vi "Initialize Buffer IDs.vi"(8 "error in":errorcluster, 10 "shared resources":refnum<class "Shared Resources.lvclass">, 11 "rx execution unit":refnum<class "Rx Execution Unit.lvclass">) -> (0 "error out":errorcluster, 3 "rx execution unit out":refnum<class "Rx Execution Unit.lvclass">)   [LabVIEW 2020, in "AIM MIL-STD-1553 Engine.lvlib" / "Implementation.lvlib" / "Rx Execution Unit.lvclass"]
uses:
  Rx Execution Unit.lvclass
  Interfaces/Shared Resources/Shared Resources.lvclass
  Shared Resources/Shared Resources.lvclass
  Shared Resources/Shared Resources.lvclass/Shared Resources.ctl
  Rx Execution Unit.lvclass/Rx Execution Unit.ctl
  Shared/Direction.ctl
  Shared Resources/Read BC Subaddress to Buffer ID Map.vi
  Shared Resources/Read RT Subaddress to Buffer ID Map.vi
  <vilib>/NI VeriStand/Custom Device Tools/Custom Device Utility Library/Custom Device Utility Library.lvlib
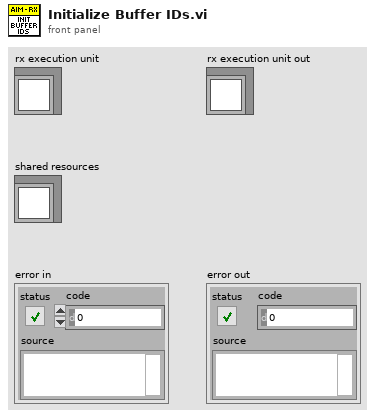
[diagram p1: front panel]
types:
  T1 = enum16{"unknown", "BC Message Buffer", "RT Message Buffer"}
  T2 = typedef "Direction.ctl" = enum16{"Rx", "Tx"}
  T3 = typedef "AIM MIL-STD-1553 Engine.lvlib/Implementation.lvlib/Shared Resources.lvclass/BC Subaddress to Buffer ID Map.ctl" = map{cluster{"TX Address":u8, "TX Subaddress":u8, "RX Address":u8, "RX Subaddress":u8}, cluster{"Buffer ID":u16}}
  T4 = typedef "AIM MIL-STD-1553 Engine.lvlib/Implementation.lvlib/Shared Resources.lvclass/RT Subaddress to Buffer ID Map.ctl" = map{cluster{"RT Address":u8, "Subaddress":u8, "Direction":T2}, cluster{"Buffer ID":u16}}
  T5 = typedef "AIM MIL-STD-1553 Engine.lvlib/Custom Device.lvlib/Compiled Message.ctl" = cluster{"Message Section Handle":T6, "First Parameter Index":i32, "Parameter Channel Handles":T6[], "Direction":T2, "Parameters":T7[], "Receiving RT Address":u8, "Receiving RT Sub-address":u8, "Transmitting RT Address":u8, "Transmitting RT Sub-address":u8, "Word Count":u8, "Buffer Type":enum16{"unknown", "BC Message Buffer", "RT Message Buffer"}, "Buffer ID":u16, "Terminal Type":enum16{"Bus Controller", "Remote Terminal"}, "Timestamp Enabled":bool, "Timestamp Channel Handle":T6}
  T6 = typedef "Custom Device API.lvlib/Custom Device Item Ref.ctl" = u64
  T7 = typedef "Parameter Definition.ctl" = cluster{"start index":i32, "size (bits)":i32, "encoding":enum16{"BNR", "BCD", "Discrete"}, "signed":bool, "multiplier":dbl, "offset":dbl}
  T8 = cluster{"Receiving RT Address":u8, "Receiving RT Sub-address":u8, "Direction":T2}
  T9 = cluster{"Transmitting RT Address":u8, "Transmitting RT Sub-address":u8, "Receiving RT Address":u8, "Receiving RT Sub-address":u8}
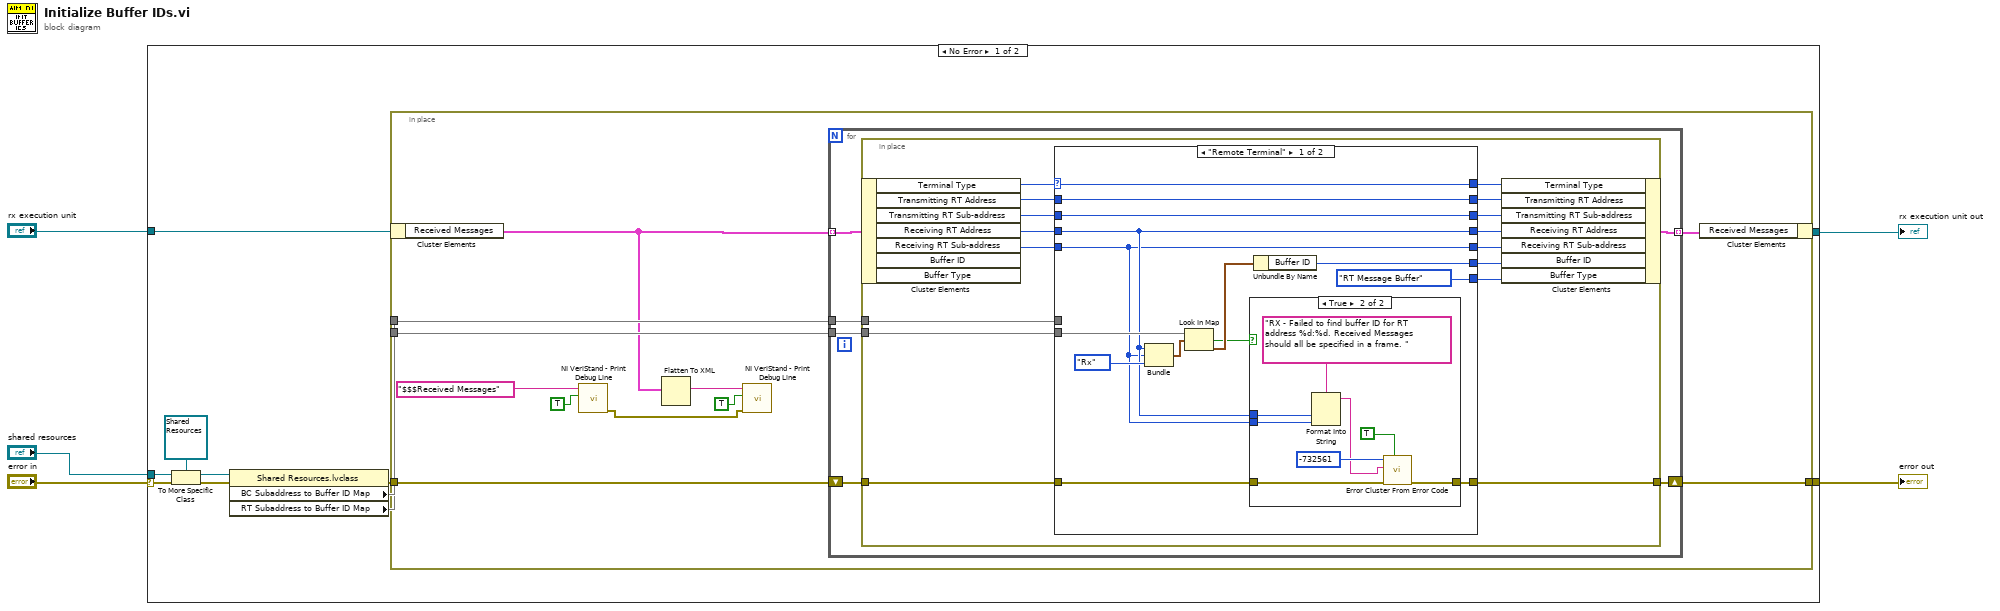
[diagram p0: block diagram]
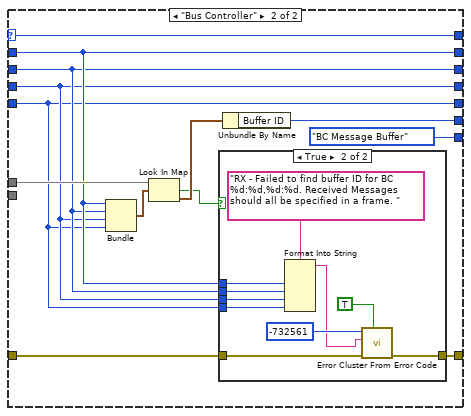
[diagram p3: hidden frame]
diagram:
  n1 = case shown="No Error" "error in" {
    selector: "error in" -> [w16 w98]
    tunnel: "shared resources" -> [w15 _]
    tunnel: [w11 w98] -> w4
    tunnel: "rx execution unit" -> [w10 w97]
    tunnel: [w9 w97] -> w2
    frame No Error {
      n2 = To More Specific Class(target class=refnum<class "Shared Resources.lvclass"> refnum ("specific class reference"), reference=w15, error in=w16) -> (specific class reference=w12:refnum<class "Shared Resources.lvclass">, error out=w6:errorcluster)
      n3 = property class="Shared Resources.lvclass"(reference=w12, error in=w6) -> (error out=w13:errorcluster, "BC Subaddress to Buffer ID Map"=w8:T3, "RT Subaddress to Buffer ID Map"=w7:T4)  [unwired: 1 out]
      n4 = in-place {
        in-place-border: w7 -> [w26]
        in-place-border: w13 -> [w25]
        in-place-border: [w24] -> w11
        in-place-border: w8 -> [w23]
        n5 = in-place-cluster #1(w10) -> ("Received Messages"=w17:T5[])
        n6 = call <vilib>:"NI VeriStand - Print Debug Line.vi"("Add to log file? (F)"=TRUE, "Message"="$$$Received Messages") -> ("error out"=w18:errorcluster)  [unwired: 9 in]
        n7 = Flatten To XML(6:w17) -> (2:w22:string)
        n8 = call <vilib>:"NI VeriStand - Print Debug Line.vi"("error in (no error)"=w18, "Add to log file? (F)"=TRUE, "Message"=w22) -> ()  [unwired: 8 in, 1 out]
        n9 = for {
          tunnel: w17 -> [w33] mode=indexing
          tunnel: [w32] -> w27 mode=indexing
          tunnel: w26 -> [w31]
          shift-right: [w29] -> w24
          shift-left: w25 -> [w30]
          tunnel: w23 -> [w28]
          n10 = in-place {
            in-place-border: w31 -> [w49]
            in-place-border: w30 -> [w48]
            in-place-border: [w47] -> w29
            in-place-border: w28 -> [w39]
            n11 = in-place-cluster #2(w33) -> ("Terminal Type"=w45:enum16{"Bus Controller", "Remote Terminal"}, "Transmitting RT Address"=w44:u8, "Transmitting RT Sub-address"=w43:u8, "Receiving RT Address"=w42:u8, "Receiving RT Sub-address"=w41:u8)  [unwired: 2 out]
            n12 = case shown="\"Remote Terminal\"" w45 {
              selector: w45 -> [w55 w79]
              tunnel: w49 -> [w62 _]
              tunnel: [w59 w83] -> w38
              tunnel: w48 -> [w57 w81]
              tunnel: [w56 w80] -> w47
              tunnel: [w55 w79] -> w46
              tunnel: w44 -> [w52 w76]
              tunnel: w43 -> [w53 w75]
              tunnel: w42 -> [w51 w74]
              tunnel: w41 -> [w50 w73]
              tunnel: [T1."RT Message Buffer" ("Buffer Type") T1."BC Message Buffer" ("Buffer Type")] -> w40
              tunnel: [w51 w74] -> w35
              tunnel: [w50 w73] -> w34
              tunnel: [w53 w75] -> w36
              tunnel: [w52 w76] -> w37
              tunnel: w39 -> [_ w77]
              frame "Remote Terminal" {
                n13 = Bundle("Receiving RT Address"=w51, "Receiving RT Sub-address"=w50, "Direction"=Direction."Rx") -> (w63:T8)  [unwired: 1 in]
                n14 = Look In Map(map=w62, key=w63) -> (key not found?=w58:bool, value=w61:cluster{"Buffer ID":u16})  [unwired: 1 in]
                n15 = case shown="True" w58 {
                  tunnel: w51 -> [_ w71]
                  tunnel: w50 -> [_ w70]
                  tunnel: w57 -> [w64 w69]
                  tunnel: [w64 w68] -> w56
                  frame False {
                  }
                  frame True {
                    n16 = Format Into String(format string="RX - Failed to find buffer ID for RT address %d:%d. Received Messages should all be specified in a frame. ", w71, w70) -> (resulting string=w66:string)  [unwired: 2 in, 1 out]
                    n17 = call <vilib>:"Error Cluster From Error Code.vi"("show call chain? (False)"=TRUE, "error in (no error)"=w69, "error message (\"\")"=w66, "error code (0)"=-732561) -> ("error out"=w68:errorcluster)  [unwired: 5 in]
                  }
                }
                n18 = Unbundle By Name(w61) -> ("Buffer ID"=w59:u16)
              }
              frame "Bus Controller" {
                n19 = Bundle("Transmitting RT Address"=w76, "Transmitting RT Sub-address"=w75, "Receiving RT Address"=w74, "Receiving RT Sub-address"=w73) -> (w85:T9)  [unwired: 1 in]
                n20 = Look In Map(map=w77, key=w85) -> (key not found?=w82:bool, value=w84:cluster{"Buffer ID":u16})  [unwired: 1 in]
                n21 = case shown="True" w82 {
                  tunnel: w76 -> [_ w95]
                  tunnel: w75 -> [_ w94]
                  tunnel: w81 -> [w86 w93]
                  tunnel: [w86 w92] -> w80
                  tunnel: w74 -> [_ w88]
                  tunnel: w73 -> [_ w87]
                  frame False {
                  }
                  frame True {
                    n22 = Format Into String(format string="RX - Failed to find buffer ID for BC %d:%d,%d:%d. Received Messages should all be specified in a frame. ", w95, w94, w88, w87) -> (resulting string=w90:string)  [unwired: 2 in, 1 out]
                    n23 = call <vilib>:"Error Cluster From Error Code.vi"("show call chain? (False)"=TRUE, "error in (no error)"=w93, "error message (\"\")"=w90, "error code (0)"=-732561) -> ("error out"=w92:errorcluster)  [unwired: 5 in]
                  }
                }
                n24 = Unbundle By Name(w84) -> ("Buffer ID"=w83:u16)
              }
            }
            n25 = in-place-cluster #2("Terminal Type"=w46, "Transmitting RT Address"=w37, "Transmitting RT Sub-address"=w36, "Receiving RT Address"=w35, "Receiving RT Sub-address"=w34, "Buffer ID"=w38, "Buffer Type"=w40) -> (w32:T5)
          }
        }
        n26 = in-place-cluster #1("Received Messages"=w27) -> (w9:refnum<class "Rx Execution Unit.lvclass">)
      }
    }
    frame Error {
    }
  }
  "error out" <- w4
  "rx execution unit out" <- w2
